vi "CompareFolderTimes.vi"(2 "SearchPath":string, 3 "Time In":timestamp) -> (1 "FolderOut":string)   [LabVIEW 2011]
uses:
  <vilib>/imath/engines/lvmath/Plug In/_Char/NIMS_CH_character datatype.ctl
  <vilib>/imath/engines/lvmath2/RunTimeEngine/ErrorHandling/NIMS_Finalize Error.vi
  <vilib>/imath/engines/lvmath2/RunTimeEngine/Managers/WorkSpace/UID Generator.vi
  <vilib>/imath/engines/lvmath/Plug In/_Char/NIMS_CH_String to Character Array.vi
  <vilib>/imath/engines/lvmath/Plug In/_Char/NIMS_CH_Character 2D to String 1D.vi
  <vilib>/imath/engines/lvmath2/RunTimeEngine/NodeEndStatement/NIMS_NodeEndStatement_Output.vi
  <instcachedir>/0/NIMS_NodeEndStatement_Output_53EC0D466D134D7ABD903AC30B43404B.lvgen/NIMS_NodeEndStatement_Output_53EC0D466D134D7ABD903AC30B43404B_006.vi
  <vilib>/imath/engines/lvmath/Plug In/_Char/NIMS_CH_Character RV to String.vi
  <vilib>/imath/engines/lvmath2/RunTimeEngine/BuiltInFunctions/pathgetsubset/NIMS_pathgetsubset(Str).vi
  <vilib>/imath/engines/lvmath2/RunTimeEngine/BuiltInFunctions/regex/NIMS_regex(Str,Str).vi
  <vilib>/imath/engines/lvmath2/RunTimeEngine/ErrorHandling/NIMS_Error From Error Code.vi
  <vilib>/imath/engines/lvmath2/RunTimeEngine/BuiltInFunctions/repeatmx/NIMS_repeatmx(GM, I32, I32).vi
  <instcachedir>/0/NIMS_repeatmx(GM, I32, I32)_8C2ED2EBCBCE41FC8E83AC0E124C0986.lvgen/NIMS_repeatmx(GM, I32, I32)_8C2ED2EBCBCE41FC8E83AC0E124C0986_004.vi
  <vilib>/imath/engines/lvmath2/RunTimeEngine/BuiltInFunctions/length/NIMS_length(GV).vi
  <instcachedir>/0/NIMS_length(GV)_08A3D13377FD4E4B96F5795FBF3698FA.lvgen/NIMS_length(GV)_08A3D13377FD4E4B96F5795FBF3698FA_002.vi
  <vilib>/imath/engines/lvmath2/RunTimeEngine/ArithmeticOperatorToken/NIMS_ArithmeticOperator_plus.vi
  <instcachedir>/0/NIMS_ArithmeticOperator_plus_1E95F7DAB906458CBECCADBE8E6FD739.lvgen/NIMS_ArithmeticOperator_plus_1E95F7DAB906458CBECCADBE8E6FD739_010.vi
  <vilib>/imath/engines/lvmath2/RunTimeEngine/ErrorHandling/NIMS_Create Error From Enums.vi
  <vilib>/imath/engines/lvmath2/RunTimeEngine/VariableToken/Read/NIMS_Get Elements - RV(_) - Check.vi
  <instcachedir>/0/NIMS_Get Elements - RV(_) - Check_B511B9D8E05044FE80F9F088FE24B20C.lvgen/NIMS_Get Elements - RV(_) - Check_B511B9D8E05044FE80F9F088FE24B20C_003.vi
  <vilib>/imath/engines/lvmath2/RunTimeEngine/BuiltInFunctions/sort/NIMS_[1o]_sort(StrV).vi
  <instcachedir>/0/NIMS_[1o]_sort(StrV)_88222AE4474142D6839FC22BD1FBF5A2.lvgen/NIMS_[1o]_sort(StrV)_88222AE4474142D6839FC22BD1FBF5A2_000.vi
  <vilib>/imath/engines/lvmath/Plug In/_Char/NIMS_CH_String CV to Character 2D.vi
  <instcachedir>/0/NIMS_CH_String CV to Character 2D_2FEA6B6DB9CD4AF49E7702F383C90008.lvgen/NIMS_CH_String CV to Character 2D_2FEA6B6DB9CD4AF49E7702F383C90008_000.vi
  <vilib>/imathl/engines/lvmath/Functions/Error Handling/Create Error.vi
panel:
  out "FolderTime":timestamp
  out "Folder":string
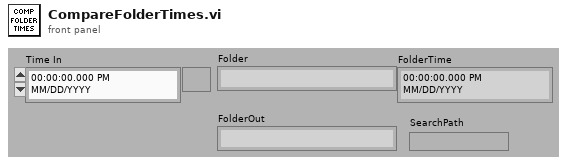
[diagram p1: front panel]
types:
  T1 = cluster{dbl, i32, i32, i32, i32, i32, i32, i32, i32, i32}
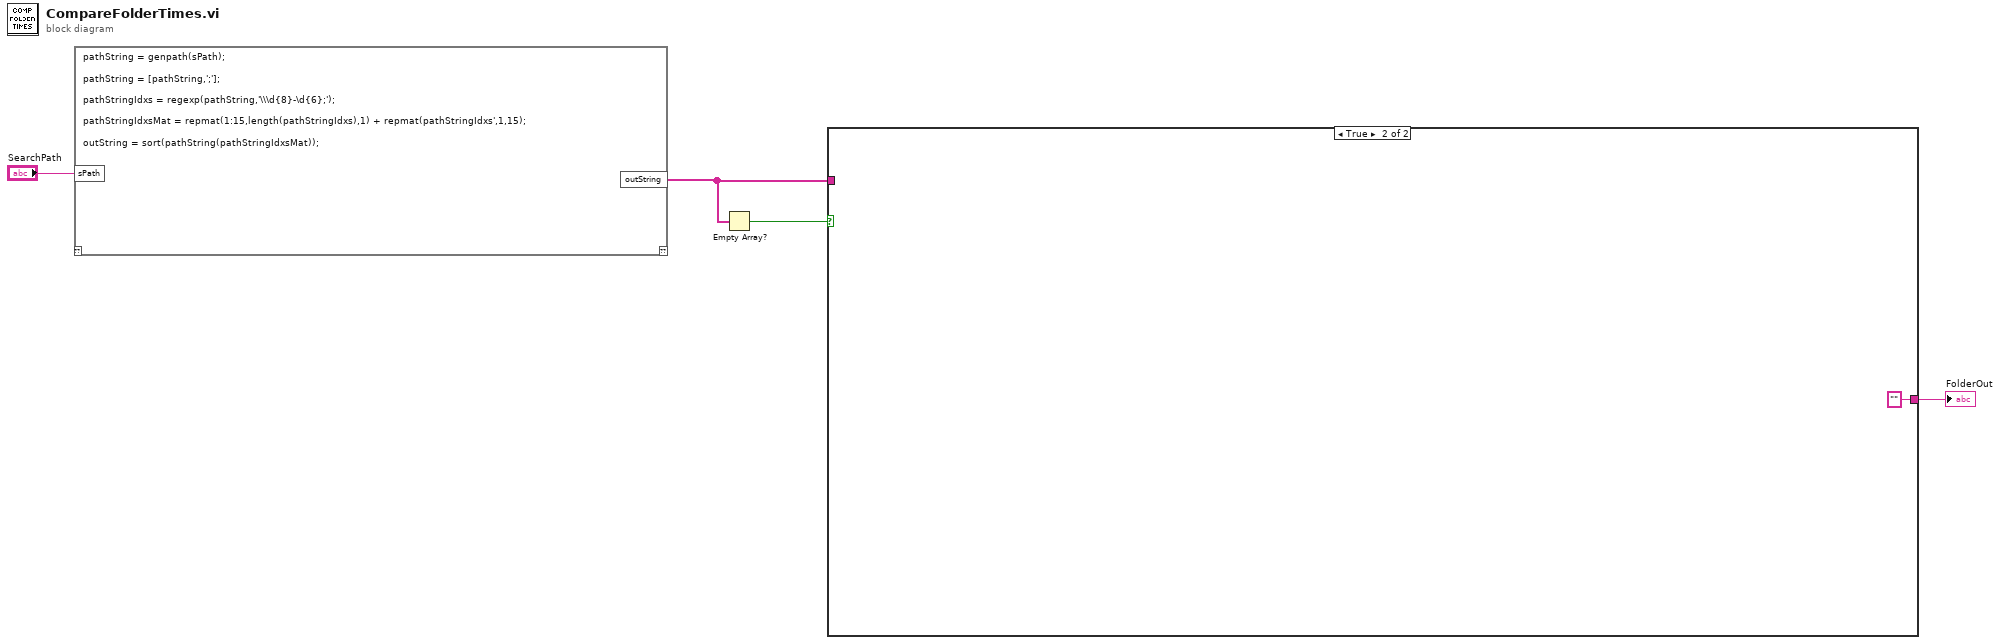
[diagram p0: block diagram]
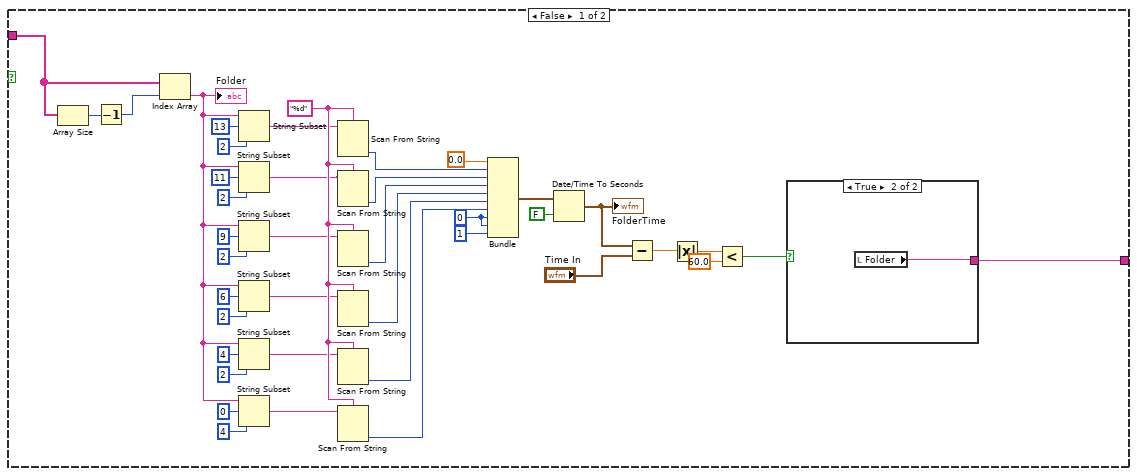
[diagram p2: hidden frame]
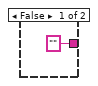
[diagram p3: hidden frame]
diagram:
  n1 = mathscript code="pathString = genpath(sPath);\n\npathString = [pathString,';'];\n\npathStringIdxs = regexp(pathString,'\\\\\\d{8}-\\d{6};');\n\npathStringIdxsMat = repmat(1:15,length(pathStringIdxs),1) + repmat(pathStringIdxs',1,15);\n\noutString = sort(pathString(pathStringIdxsMat));"("sPath"="SearchPath") -> ("outString"=w4:string[])  [unwired: 1 in, 1 out]
  n2 = Empty Array?(array=w4) -> (empty?=w1:bool)
  n3 = case shown="True" w1 {
    tunnel: w4 -> [w6 _]
    tunnel: [w5 "" ("Folder 1")] -> w2
    frame False {
      w42 = 0
      w32 = "%d" ("format string")
      n4 = Array Size(array=w6) -> (size(s)=w44:i32)
      n5 = Decrement(x=w44) -> (x-1=w45:i32)
      n6 = Index Array(array=w6, index=w45) -> (element=w13:string)
      "Folder" <- w13
      n7 = String Subset(string=w13, offset (0)=13, length (rest)=2 ("length (rest)")) -> (substring=w26:string)
      n8 = String Subset(string=w13, offset (0)=11, length (rest)=2 ("length (rest)")) -> (substring=w27:string)
      n9 = String Subset(string=w13, offset (0)=9, length (rest)=2 ("length (rest)")) -> (substring=w28:string)
      n10 = String Subset(string=w13, offset (0)=6, length (rest)=2 ("length (rest)")) -> (substring=w29:string)
      n11 = String Subset(string=w13, offset (0)=4, length (rest)=2 ("length (rest)")) -> (substring=w30:string)
      n12 = String Subset(string=w13, offset (0)=0, length (rest)=4 ("length (rest)")) -> (substring=w31:string)
      n13 = Scan From String(format string=w32, input string=w26) -> (output 1=w33:i32)  [unwired: 3 in, 3 out]
      n14 = Scan From String(format string=w32, input string=w27) -> (output 1=w34:i32)  [unwired: 3 in, 3 out]
      n15 = Scan From String(format string=w32, input string=w28) -> (output 1=w35:i32)  [unwired: 3 in, 3 out]
      n16 = Scan From String(format string=w32, input string=w29) -> (output 1=w36:i32)  [unwired: 3 in, 3 out]
      n17 = Scan From String(format string=w32, input string=w30) -> (output 1=w37:i32)  [unwired: 3 in, 3 out]
      n18 = Scan From String(format string=w32, input string=w31) -> (output 1=w38:i32)  [unwired: 3 in, 3 out]
      n19 = Bundle(0.0, w33, w34, w35, w36, w37, w38, w42, w42, 1) -> (w41:T1)  [unwired: 1 in]
      n20 = Date/Time To Seconds(1:FALSE ("is UTC (F)"), 2:w41) -> (0:w12:timestamp)
      "FolderTime" <- w12
      n21 = Subtract(x=w12, y="Time In") -> (x-y=w10:dbl)
      n22 = Absolute Value(x=w10) -> (abs(x)=w9:dbl)
      n23 = Less?(x=w9, y=60.0) -> (x < y?=w7:bool)
      n24 = case shown="True" w7 {
        tunnel: ["" ("Folder 1") w47] -> w5
        frame False {
        }
        frame True {
          n25 = local read "Folder"() -> (w47:string)
        }
      }
    }
    frame True {
    }
  }
  "FolderOut" <- w2
